vi "ReadSerialNumber.vi"(8 "error in (no error)":errorcluster, 11 "TestBench in":refnum<class "TestBench.lvclass">) -> (0 "error out":errorcluster, 3 "TestBench out":refnum<class "TestBench.lvclass">)   [LabVIEW 2019, in "TestBench.lvlib" / "TestBench.lvclass"]
uses:
  TestBench.lvclass
  TestBench.lvclass/TestBench.ctl
  TestEngine/TestEngine Messages/Write SerialNumber Msg/Write SerialNumber Msg.lvclass/Write SerialNumber Msg.ctl
  <vilib>/ActorFramework/Message Enqueuer/Message Enqueuer.lvclass/Message Enqueuer.ctl
  <vilib>/ActorFramework/Message Enqueuer/Enqueue.vi
  TestEngine/TestEngine Messages/Write SerialNumber Msg/Write SerialNumber Msg.lvclass
  C:/Program Files (x86)/National Instruments/LabVIEW 2019/vi.lib/ActorFramework/Message/Message.lvclass
  <vilib>/ActorFramework/Message Priority Queue/Priority Enqueue.vi
panel:
  in  "Cancel":bool
  in  "SerialNumber":string
  in  "OK":bool
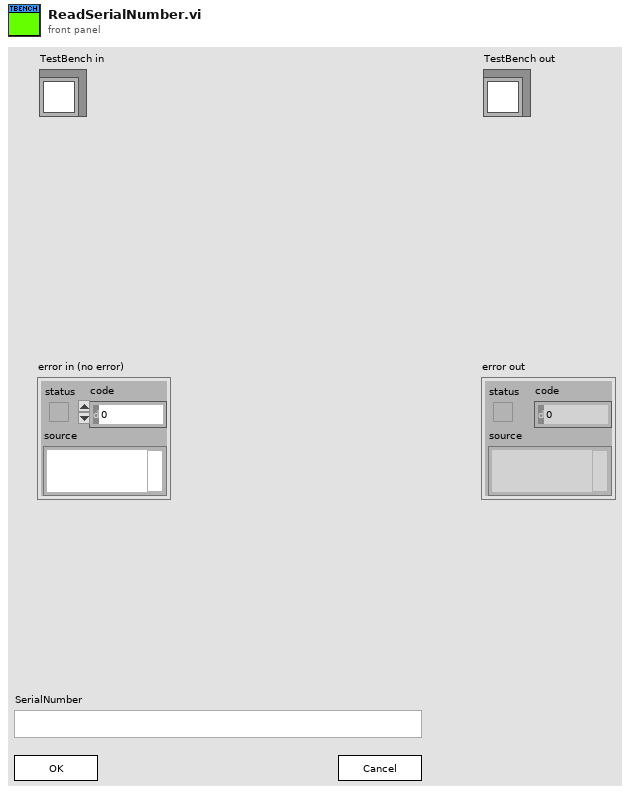
[diagram p1: front panel]
types:
  T1 = map{string, refnum<class "Message Enqueuer.lvclass">}
  T2 = cluster{string, "TestEngine Actor's Enqueuer":refnum<class "Message Enqueuer.lvclass">}
  T3 = enum32{"Invalid", "Standard", "Closed", "Hidden", "Minimized", "Maximized"}
  T4 = enum32{"invalid app kind", "Development System", "Run Time System", "Student Edition", "Embedded LabVIEW", "Evaluation", "Custom"}
  T5 = cluster{"Core":cluster{"Current VI Reference":refnum<vi>, "Close Panel on Exit?":bool}, "Your string data":string, "SerialNumber":refnum<vi>}
  T6 = cluster{"Current VI Reference":refnum<vi>, "Close Panel on Exit?":bool}
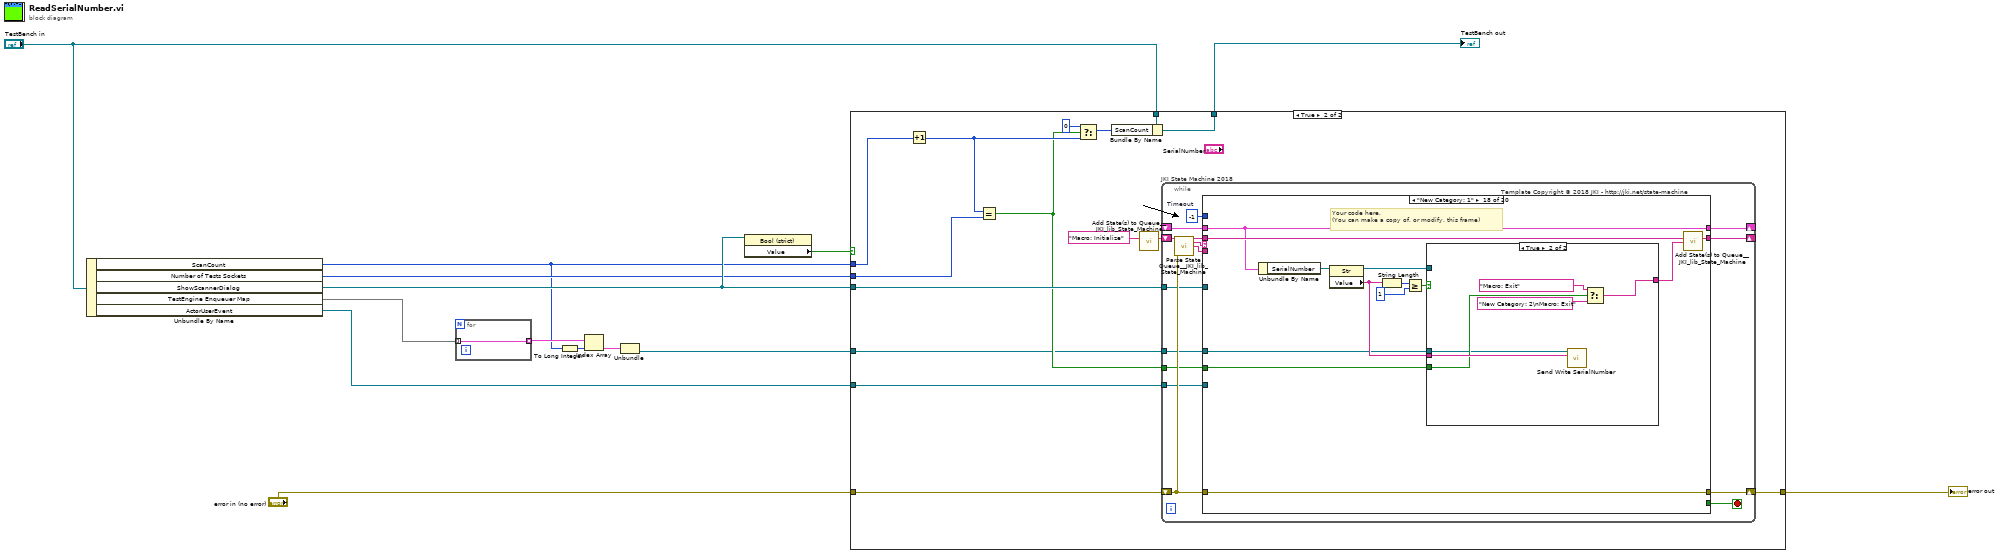
[diagram p0: block diagram]
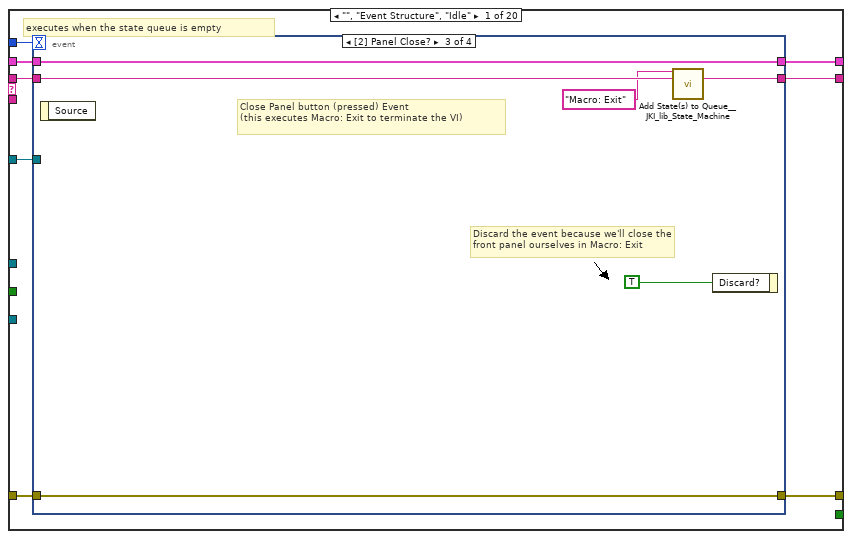
[diagram p3: hidden frame]
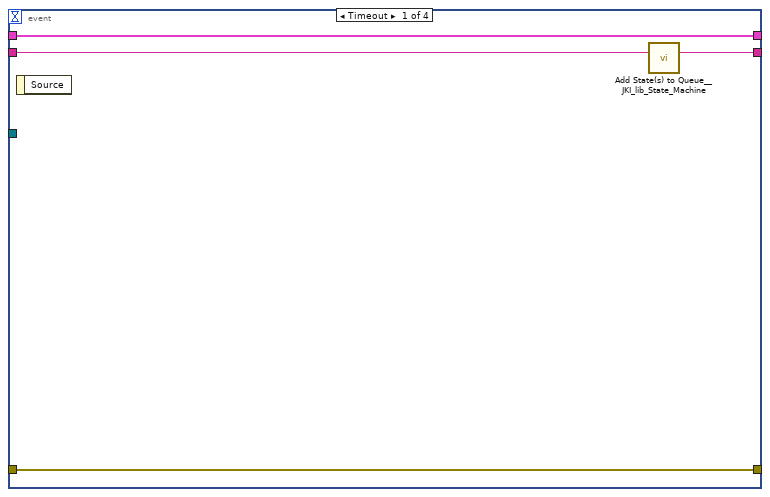
[diagram p4: hidden frame]
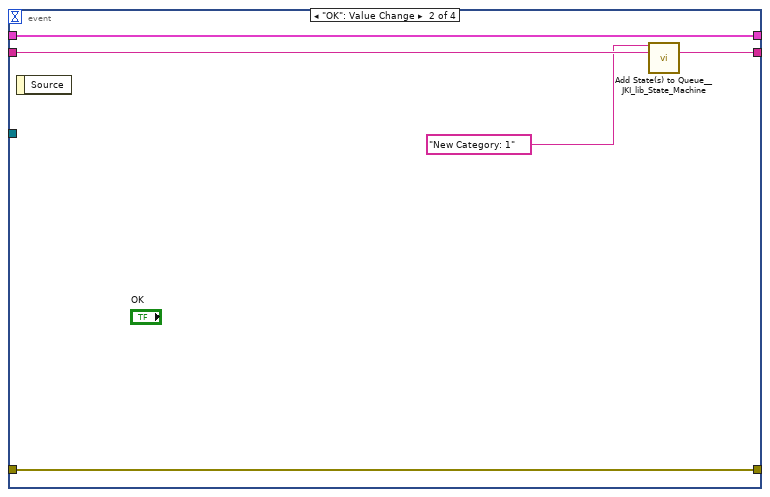
[diagram p5: hidden frame]
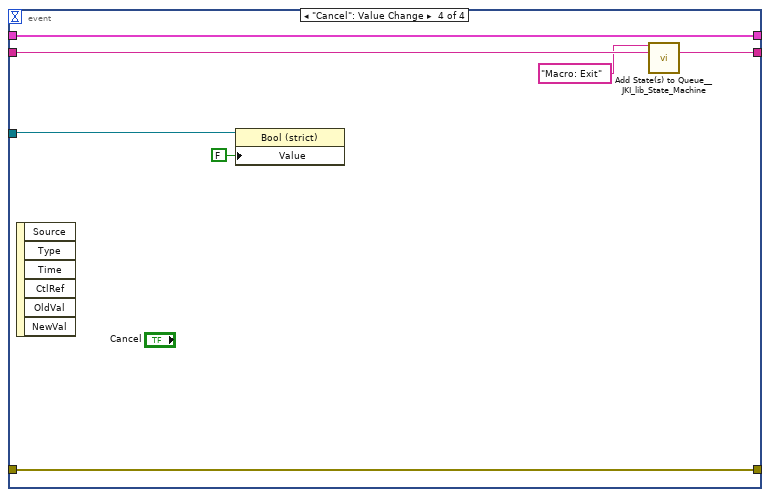
[diagram p6: hidden frame]
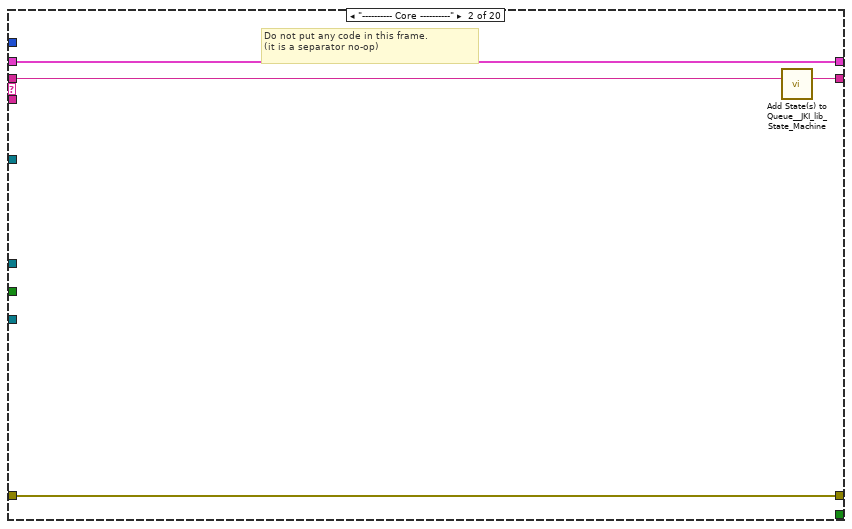
[diagram p7: hidden frame]
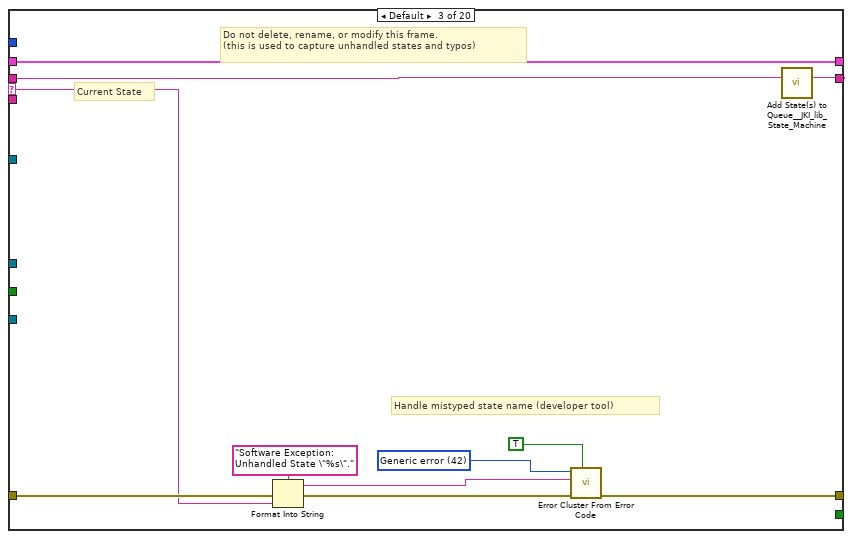
[diagram p8: hidden frame]
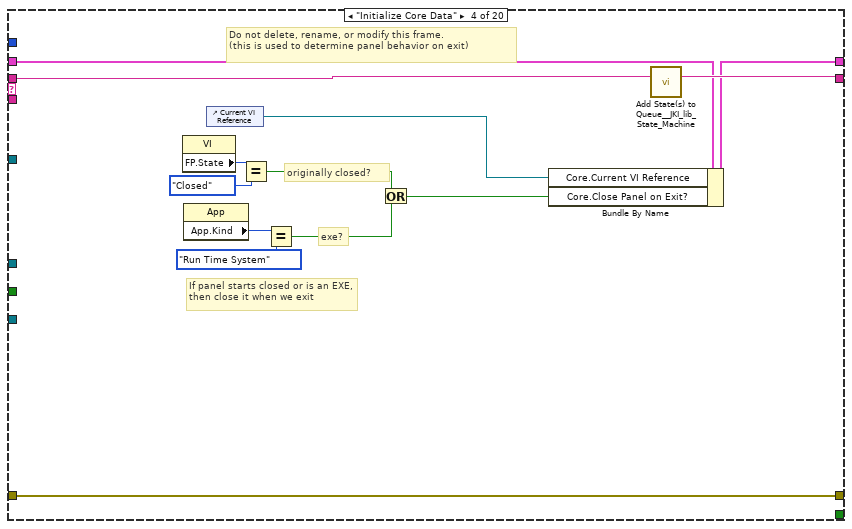
[diagram p9: hidden frame]
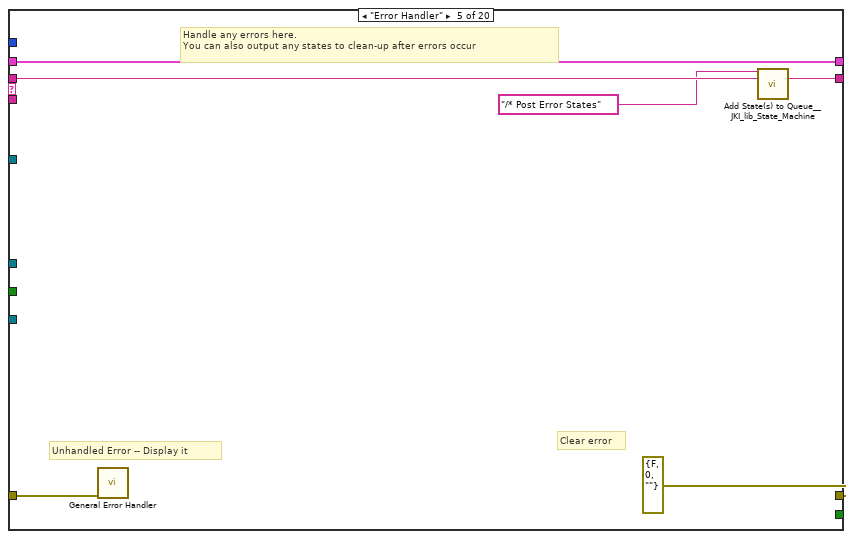
[diagram p10: hidden frame]
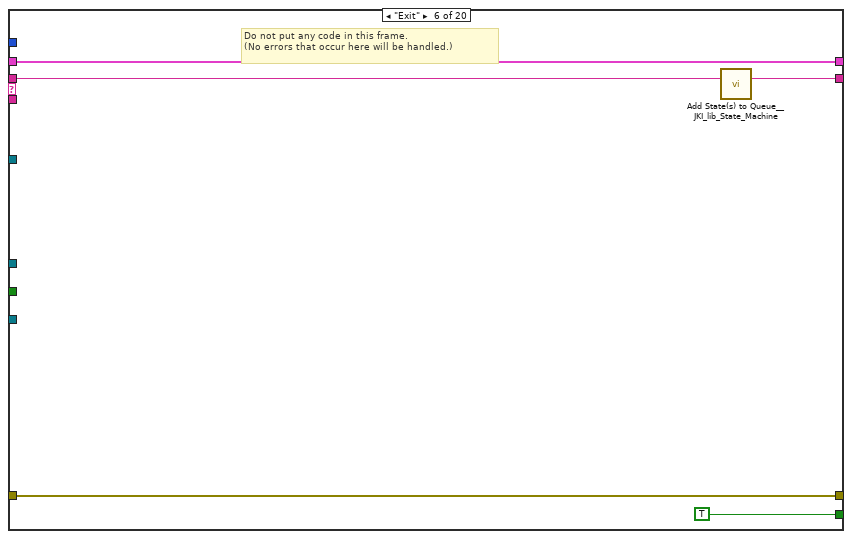
[diagram p11: hidden frame]
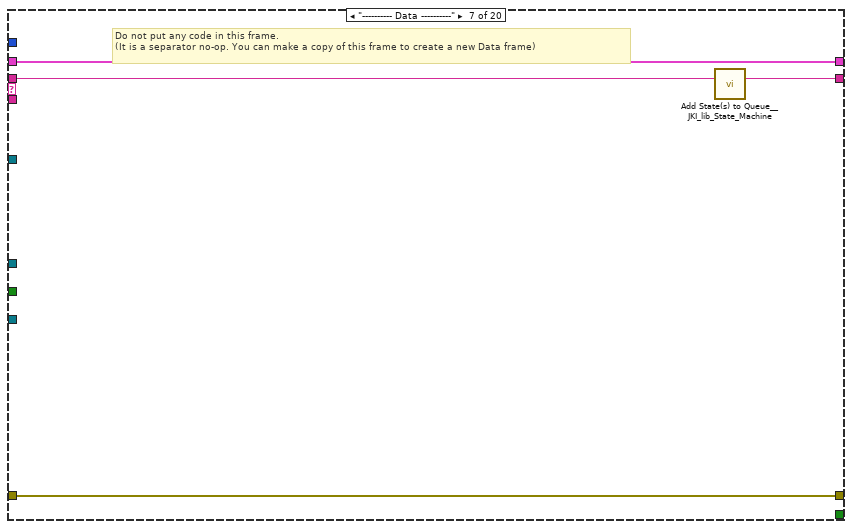
[diagram p12: hidden frame]
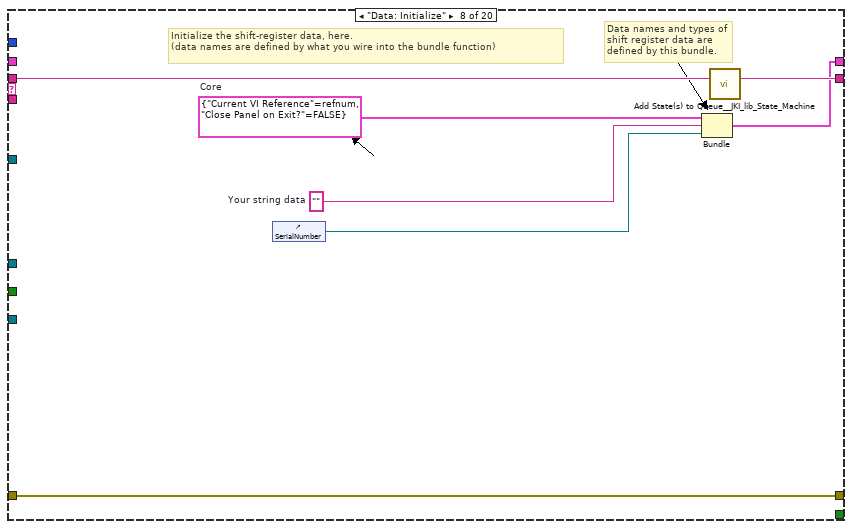
[diagram p13: hidden frame]
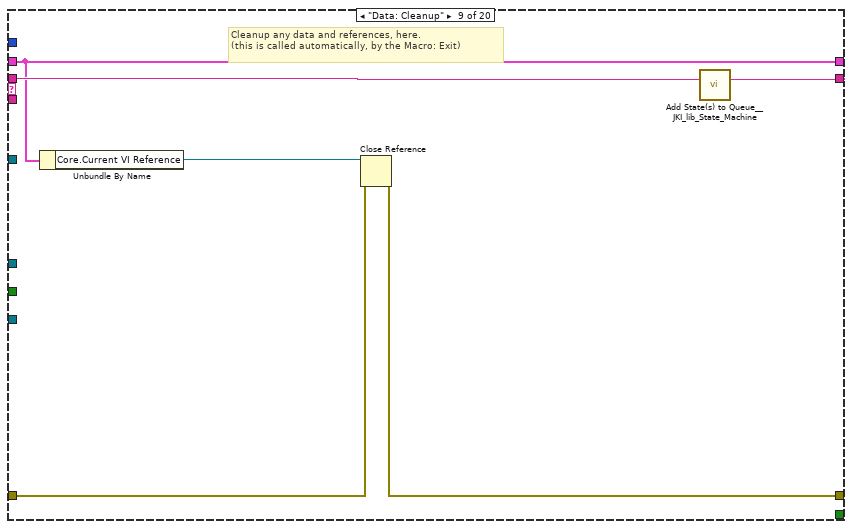
[diagram p14: hidden frame]
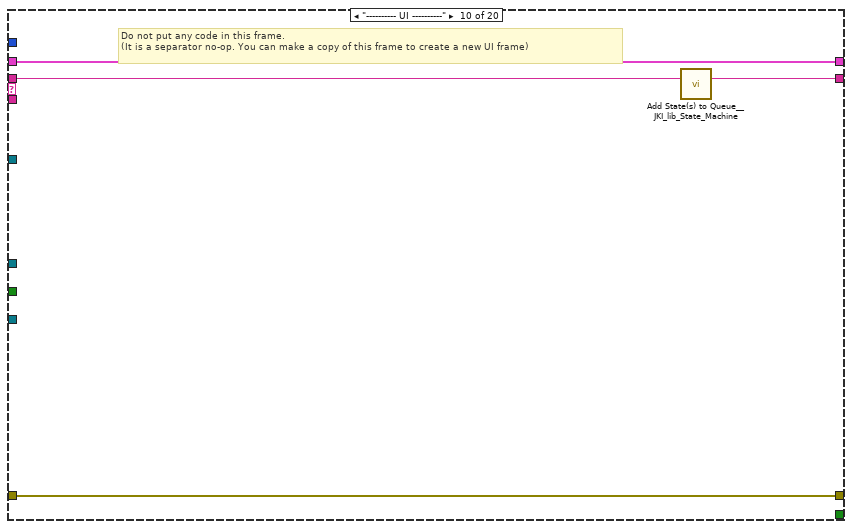
[diagram p15: hidden frame]
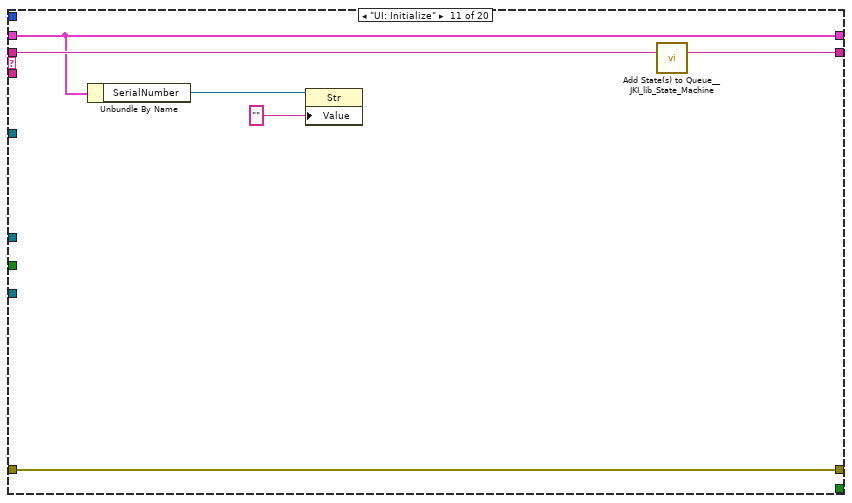
[diagram p16: hidden frame]
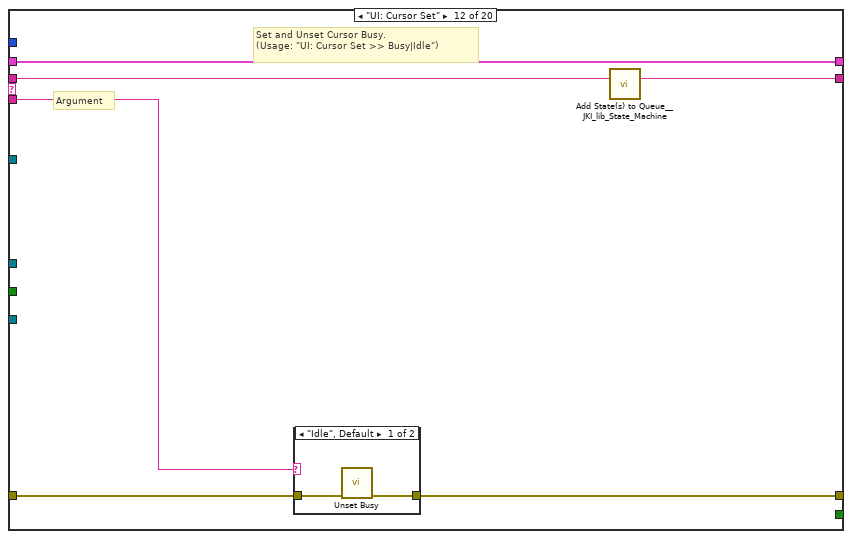
[diagram p17: hidden frame]
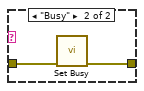
[diagram p18: hidden frame]
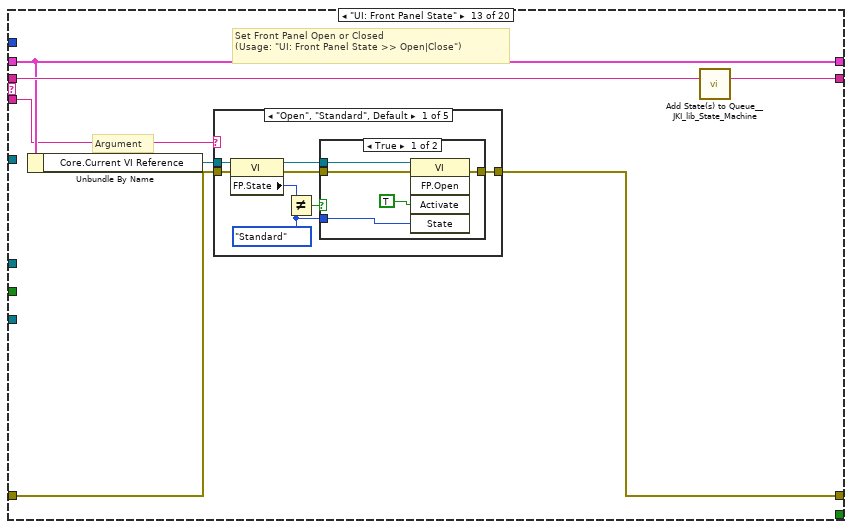
[diagram p19: hidden frame]
diagram:
  n1 = Unbundle By Name("TestBench in") -> ("ScanCount"=w4:u8, "Number of Tests Sockets"=w9:u8, "ShowScannerDialog"=w11:refnum<vi>, "TestEngine Enqueuer Map"=w6:T1, "ActorUserEvent"=w10:refnum<user-event>)
  n2 = for {
    tunnel: [w15] -> w5 mode=indexing
    tunnel: w6 -> [w15] mode=indexing
  }
  n3 = To Long Integer(number=w4) -> (32bit integer=w3:i32)
  n4 = Index Array(array=w5, index=w3) -> (element=w2:T2)
  n5 = Unbundle(w2) -> ("TestEngine Actor's Enqueuer"=w1:refnum<class "Message Enqueuer.lvclass">)  [unwired: 1 out]
  n6 = property class="Bool (strict)"(reference=w11) -> ("Value"=w12:bool)  [unwired: 1 in, 2 out]
  n7 = case shown="True" w12 {
    tunnel: "error in (no error)" -> [w17 w30]
    tunnel: [w17 w29] -> w13
    tunnel: w11 -> [_ w28]
    tunnel: w10 -> [_ w27]
    tunnel: w4 -> [_ w24]
    tunnel: w9 -> [_ w23]
    tunnel: "TestBench in" -> [w16 w20]
    tunnel: [w16 w19] -> w7
    tunnel: w1 -> [_ w18]
    frame False {
    }
    frame True {
      n8 = Increment(x=w24) -> (x+1=w26:u8)
      n9 = Equal?(x=w26, y=w23) -> (x = y?=w22:bool)
      n10 = Select(t=u8 0, s=w22, f=w26) -> (s? t:f=w21:u8)
      n11 = Bundle By Name(cluster=w20, "ScanCount"=w21) -> (w19:refnum<class "TestBench.lvclass">)
      n12 = call <vilib>:"Add State(s) to Queue__JKI_lib_State_Machine.vi"("State(s) in (\"\")"="Macro: Initialize") -> ("States Out"=w32:string)  [unwired: 14 in]
      n13 = while "JKI State Machine 2018" {
        shift-right: [w40] -> _
        shift-left: _ -> [w39]
        shift-right: [w43] -> w29
        shift-left: w30 -> [w37]
        shift-right: [w42] -> _
        shift-left: w32 -> [w44]
        tunnel: w28 -> [w36]
        tunnel: w27 -> [w35]
        tunnel: w22 -> [w34]
        tunnel: w18 -> [w33]
        stop <- w41 stop-if-true
        w38 = -1  # Timeout
        # "Template Copyright © 2018 JKI - http://jki.net/state-machine"
        n14 = call <vilib>:"Parse State Queue__JKI_lib_State_Machine.vi"("State Queue"=w44, "Error In (no error)"=w37) -> ("Remaining States"=w46:string, "Current State"=w47:string, "Arguments"=w45:string)  [unwired: 11 in]
        n15 = case shown="\"New Category: 1\"" w47 {
          selector: w47 -> [_ _ w82 _ _ _ _ _ _ _ _ _ _ _ _ _ _ _ _ _]
          tunnel: w46 -> [w55 w81 w86 w105 w111 w116 w120 w127 w133 w137 w143 w149 w160 w229 w234 w244 w248 w261 w279 w285]
          tunnel: w45 -> [_ _ _ _ _ _ _ _ _ _ _ w144 w154 _ _ _ _ _ _ _]
          tunnel: w39 -> [w53 w78 w84 w98 w108 w114 w117 _ w128 w134 w138 w147 w156 w226 w231 w241 w245 w258 w276 w281]
          tunnel: [w52 w79 w88 w102 errorcluster {"status"=FALSE, "code"=0, "source"=""} ("error out") w113 w118 w124 w129 w135 w141 w145 w157 w227 w232 w242 w246 w259 w277 w283] -> w43
          tunnel: w37 -> [w51 w79 w87 w102 w107 w113 w118 w124 w130 w135 w141 w146 w158 w227 w232 w242 w246 w259 w277 w283]
          tunnel: [w54 w80 w85 w104 w110 w115 w119 w126 w132 w136 w142 w148 w159 w228 w233 w243 w247 w260 w278 w284] -> w42
          tunnel: [_ _ _ _ _ TRUE _ _ _ _ _ _ _ _ _ _ _ _ _ _] -> w41
          tunnel: [w50 w78 w84 w103 w108 w114 w117 w125 w128 w134 w138 w147 w156 w226 w231 w241 w245 w258 w276 w281] -> w40
          tunnel: w38 -> [w49 _ _ _ _ _ _ _ _ _ _ _ _ _ _ _ _ _ _ _]
          tunnel: w36 -> [w48 _ _ _ _ _ _ _ _ _ _ _ _ _ _ _ _ _ _ _]
          tunnel: w35 -> [_ _ _ _ _ _ _ _ _ _ _ _ _ _ _ _ _ _ w275 _]
          tunnel: w34 -> [_ _ _ _ _ _ _ _ _ _ _ _ _ _ _ _ _ w251 _ _]
          tunnel: w33 -> [_ _ _ _ _ _ _ _ _ _ _ _ _ _ _ _ _ w249 _ _]
          frame "", "Event Structure", "Idle" {
            # "executes when the state queue is empty"
            n16 = event shown="[2] Panel Close?" {
              selector: _ -> [_ _ _ _]
              dyn-events: _ -> [_ _ _ _]
              timeout: w49 -> [_ _ _ _]
              tunnel: w55 -> [w59 w64 w70 w77]
              tunnel: [w58 w63 w69 w76] -> w54
              tunnel: w53 -> [w56 w61 w67 w74]
              tunnel: [w57 w62 w68 w75] -> w52
              tunnel: w51 -> [w57 w62 w68 w75]
              tunnel: [w56 w61 w67 w74] -> w50
              tunnel: w48 -> [_ _ _ w72]
              event Timeout {
                n17 = event-data() -> ()  [unwired: 1 in, 1 out]
                n18 = call <vilib>:"Add State(s) to Queue__JKI_lib_State_Machine.vi"("State(s) in (\"\")"=w59) -> ("States Out"=w58:string)  [unwired: 14 in]
              }
              event "OK": Value Change {
                n19 = event-data() -> ()  [unwired: 1 in, 1 out]
                n20 = call <vilib>:"Add State(s) to Queue__JKI_lib_State_Machine.vi"("State(s) in Front (\"\")"="New Category: 1", "State(s) in (\"\")"=w64) -> ("States Out"=w63:string)  [unwired: 13 in]
              }
              event Panel Close? {
                # "Discard the event because we'll close the front panel ourselves in Macro: Exit"
                # "Close Panel button (pressed) Event\n(this executes Macro: Exit to terminate the VI)"
                n21 = event-data() -> ()  [unwired: 1 in, 1 out]
                n22 = call <vilib>:"Add State(s) to Queue__JKI_lib_State_Machine.vi"("State(s) in Front (\"\")"="Macro: Exit", "State(s) in (\"\")"=w70) -> ("States Out"=w69:string)  [unwired: 13 in]
                n23 = event-data("Discard?"=TRUE) -> ()  [unwired: 1 in, 1 out]
              }
              event "Cancel": Value Change {
                n24 = event-data() -> ()  [unwired: 1 in, 6 out]
                n25 = property class="Bool (strict)"(reference=w72, "Value"=FALSE) -> ()  [unwired: 1 in, 2 out]
                n26 = call <vilib>:"Add State(s) to Queue__JKI_lib_State_Machine.vi"("State(s) in Front (\"\")"="Macro: Exit", "State(s) in (\"\")"=w77) -> ("States Out"=w76:string)  [unwired: 13 in]
              }
            }
          }
          frame "---------- Core ----------" {
            # "Do not put any code in this frame.\n(it is a separator no-op)"
            n27 = call <vilib>:"Add State(s) to Queue__JKI_lib_State_Machine.vi"("State(s) in (\"\")"=w81) -> ("States Out"=w80:string)  [unwired: 14 in]
          }
          frame Default {
            w91 = 42 items=["No error", "Argument error", "Memory is full", "Out of zone", "End of file", "File already open", "Generic file I/O error", "File not found", "File permission error", "Disk is full", "Duplicate path", "Too many files open", "System feature not enabled", "Resource file not found", "Cannot add resource", "Resource not found", "Image not found", "Image memory error", "Pen does not exist", "Config type invalid", "Config token not found", "Config parse error", "Config memory error", "Bad external code format", "Bad external code offset", "External code not present", "Null window", "Destroy window error", "Null menu", "Print aborted", "Bad print record", "Print driver error", "Windows error during printing", "Memory error during printing", "Print dialog error", "Generic print error", "Invalid device refnum", "Device not found", "Device parameter error", "Device unit error", "Cannot open device", "Device call aborted", "Generic error", "Cancelled by user", "Object ID too low", "Object ID too high", "Object not in heap", "Unknown heap", "Unknown object (invalid DefProc)", "Unknown object (DefProc not in table)", "Message out of range", "Invalid (null) method", "Unknown message", "Manager call not supported", "Bad address", "Network operation in progress", "Network operation timed out", "Connection is busy", "Network attribute not supported", "Network error", "Address in use", "System out of memory", "Connection aborted", "Connection refused", "Not connected", "Already connected", "Connection closed", "Initialization error (interapplication manager)", "Bad occurrence", "Wait on unbound occurrence handler", "Occurrence queue overflow", "Datalog type conflict", "Unused", "Unrecognized type (interapplication manager)", "Memory corrupt", "Failed to make temporary DLL", "Old CIN version", "Drag socket not found", "Failed to load drop-object", "Failed to register OLE object", "Failed to release OLE object", "Format specifier type mismatch", "Unknown format specifier", "Too few format specifiers", "Too many format specifiers", "Scan failed", "Newer CIN version", "Error converting to variant", "Runtime menu error", "Password tampered", "Variant attribute not found", "Incompatible variant data type", "Event data is not available", "Event Store is not present", "Occurrence is not found", "Event Queue is not created", "Event info is not available", "Refnum passed is NULL", "Error retrieving Class GUID", "Error retrieving CoClass GUID", "Error retrieving TypeLib GUID.", "Bad built application magic bytes.", "Specific driver is different from the specific driver associated with the Logical Name.", "There is no session opened to the class driver.", "Max Error", "MAX - Error with config objects", "MAX - Error loading configuration", "MAX - Group not supported"]
            # "Current State"
            # "Do not delete, rename, or modify this frame.\n(this is used to capture unhandled states and typos)"
            # "Handle mistyped state name (developer tool)"
            n28 = Format Into String(format string="Software Exception: Unhandled State \"%s\"." ("message"), error in=w87, w82) -> (resulting string=w90:string, error out=w89:errorcluster)  [unwired: 1 in]
            n29 = call <vilib>:"Error Cluster From Error Code.vi"("show call chain? (False)"=TRUE, "error in (no error)"=w89, "error message (\"\")"=w90, "error code (0)"=w91) -> ("error out"=w88:errorcluster)  [unwired: 5 in]
            n30 = call <vilib>:"Add State(s) to Queue__JKI_lib_State_Machine.vi"("State(s) in (\"\")"=w86) -> ("States Out"=w85:string)  [unwired: 14 in]
          }
          frame "Initialize Core Data" {
            # "Do not delete, rename, or modify this frame.\n(this is used to determine panel behavior on exit)"
            # "originally closed?"
            # "exe?"
            # "If panel starts closed or is an EXE, then close it when we exit"
            n31 = property class="VI"() -> ("FP.State"=w95:T3)  [unwired: 2 in, 2 out]
            n32 = property class="App"() -> ("App.Kind"=w101:T4)  [unwired: 2 in, 2 out]
            n33 = control-ref of="Current VI Reference"() -> (w96:refnum<vi>)
            n34 = Equal?(x=w95, y=T3."Closed" ("Front Panel Window:State")) -> (x = y?=w93:bool)
            n35 = Equal?(x=w101, y=T4."Run Time System" ("Application:Kind")) -> (x = y?=w99:bool)
            n36 = Or(x=w93, y=w99) -> (x .or. y?=w97:bool)
            n37 = Bundle By Name(cluster=w98, "Core.Current VI Reference"=w96, "Core.Close Panel on Exit?"=w97) -> (w103:T5)
            n38 = call <vilib>:"Add State(s) to Queue__JKI_lib_State_Machine.vi"("State(s) in (\"\")"=w105) -> ("States Out"=w104:string)  [unwired: 14 in]
          }
          frame "Error Handler" {
            # "Unhandled Error -- Display it"
            # "Handle any errors here.\nYou can also output any states to clean-up after errors occur"
            # "Clear error"
            n39 = call <vilib>:"General Error Handler.vi"("error in (no error)"=w107) -> ()  [unwired: 10 in, 5 out]
            n40 = call <vilib>:"Add State(s) to Queue__JKI_lib_State_Machine.vi"("State(s) in Front (\"\")"="/* Post Error States", "State(s) in (\"\")"=w111) -> ("States Out"=w110:string)  [unwired: 13 in]
          }
          frame "Exit" {
            # "Do not put any code in this frame.\n(No errors that occur here will be handled.)"
            n41 = call <vilib>:"Add State(s) to Queue__JKI_lib_State_Machine.vi"("State(s) in (\"\")"=w116) -> ("States Out"=w115:string)  [unwired: 14 in]
          }
          frame "---------- Data ----------" {
            # "Do not put any code in this frame.\n(It is a separator no-op. You can make a copy of this frame to create a new Data frame)"
            n42 = call <vilib>:"Add State(s) to Queue__JKI_lib_State_Machine.vi"("State(s) in (\"\")"=w120) -> ("States Out"=w119:string)  [unwired: 14 in]
          }
          frame "Data: Initialize" {
            w123 = T6 {"Current VI Reference"=refnum, "Close Panel on Exit?"=FALSE}  # Core
            w121 = ""  # Your string data
            # "Data names and types of shift register data are defined by this bundle."
            # "Initialize the shift-register data, here.\n(data names are defined by what you wire into the bundle function)"
            n43 = control-ref of="SerialNumber"() -> (w122:refnum<vi>)
            n44 = Bundle("Core"=w123, "Your string data"=w121, "SerialNumber"=w122) -> (w125:T5)  [unwired: 1 in]
            n45 = call <vilib>:"Add State(s) to Queue__JKI_lib_State_Machine.vi"("State(s) in (\"\")"=w127) -> ("States Out"=w126:string)  [unwired: 14 in]
          }
          frame "Data: Cleanup" {
            # "Cleanup any data and references, here.\n(this is called automatically, by the Macro: Exit)"
            n46 = Unbundle By Name(w128) -> ("Core.Current VI Reference"=w131:refnum<vi>)
            n47 = Close Reference(reference=w131, error in (no error)=w130) -> (error out=w129:errorcluster)
            n48 = call <vilib>:"Add State(s) to Queue__JKI_lib_State_Machine.vi"("State(s) in (\"\")"=w133) -> ("States Out"=w132:string)  [unwired: 14 in]
          }
          frame "---------- UI ----------" {
            # "Do not put any code in this frame.\n(It is a separator no-op. You can make a copy of this frame to create a new UI frame)"
            n49 = call <vilib>:"Add State(s) to Queue__JKI_lib_State_Machine.vi"("State(s) in (\"\")"=w137) -> ("States Out"=w136:string)  [unwired: 14 in]
          }
          frame "UI: Initialize" {
            n50 = Unbundle By Name(w138) -> ("SerialNumber"=w140:refnum<vi>)
            n51 = property class="Str"(reference=w140, "Value"="") -> ()  [unwired: 1 in, 2 out]
            n52 = call <vilib>:"Add State(s) to Queue__JKI_lib_State_Machine.vi"("State(s) in (\"\")"=w143) -> ("States Out"=w142:string)  [unwired: 14 in]
          }
          frame "UI: Cursor Set" {
            # "Argument"
            # "Set and Unset Cursor Busy.\n(Usage: \"UI: Cursor Set >> Busy|Idle\")"
            n53 = case shown="\"Idle\", Default" w144 {
              tunnel: w146 -> [w151 w153]
              tunnel: [w150 w152] -> w145
              frame "Idle", Default {
                n54 = call <vilib>:"Unset Busy.vi"("error in (no error)"=w151) -> ("error out"=w150:errorcluster)  [unwired: 10 in]
              }
              frame "Busy" {
                n55 = call <vilib>:"Set Busy.vi"("error in (no error)"=w153) -> ("error out"=w152:errorcluster)  [unwired: 9 in, 1 out]
              }
            }
            n56 = call <vilib>:"Add State(s) to Queue__JKI_lib_State_Machine.vi"("State(s) in (\"\")"=w149) -> ("States Out"=w148:string)  [unwired: 14 in]
          }
          frame "UI: Front Panel State" {
            # "Argument"
            # "Set Front Panel Open or Closed\n(Usage: \"UI: Front Panel State >> Open|Close\")"
            n57 = Unbundle By Name(w156) -> ("Core.Current VI Reference"=w155:refnum<vi>)
            n58 = case shown="\"Open\", \"Standard\", Default" w154 {
              tunnel: w158 -> [w166 w181 w192 w205 w218]
              tunnel: [w168 w182 w194 w207 w220] -> w157
              tunnel: w155 -> [w167 w179 w193 w206 w219]
              frame "Open", "Standard", Default {
                w161 = T3."Standard" ("State")
                n59 = property class="VI"(reference=w167, error in=w166) -> (reference out=w164:refnum<vi>, error out=w165:errorcluster, "FP.State"=w163:T3)
                n60 = Not Equal?(x=w163, y=w161) -> (x != y?=w162:bool)
                n61 = case shown="True" w162 {
                  tunnel: [w172 w174] -> w168
                  tunnel: w165 -> [w171 w174]
                  tunnel: w164 -> [w170 _]
                  tunnel: w161 -> [w169 _]
                  frame True {
                    n62 = invoke class="VI" method="FP.Open"(reference=w170, error in=w171, "Activate"=TRUE, "State"=w169) -> (error out=w172:errorcluster)  [unwired: 1 in, 4 out]
                  }
                  frame False {
                  }
                }
              }
              frame "Close", "Closed" {
                n63 = property class="VI"(reference=w179, error in=w181) -> (reference out=w178:refnum<vi>, error out=w180:errorcluster, "FP.State"=w176:T3)
                n64 = Not Equal?(x=w176, y=T3."Closed" ("Front Panel Window:State")) -> (x != y?=w175:bool)
                n65 = case shown="True" w175 {
                  tunnel: [w183 w186] -> w182
                  tunnel: w180 -> [w183 w185]
                  tunnel: w178 -> [_ w184]
                  frame False {
                  }
                  frame True {
                    n66 = invoke class="VI" method="FP.Close"(reference=w184, error in=w185) -> (error out=w186:errorcluster)  [unwired: 1 in, 2 out]
                  }
                }
              }
              frame "Hidden", "Hide" {
                w187 = T3."Hidden" ("State")
                n67 = property class="VI"(reference=w193, error in=w192) -> (reference out=w190:refnum<vi>, error out=w191:errorcluster, "FP.State"=w189:T3)
                n68 = Not Equal?(x=w189, y=w187) -> (x != y?=w188:bool)
                n69 = case shown="True" w188 {
                  tunnel: [w198 w199] -> w194
                  tunnel: w191 -> [w197 w199]
                  tunnel: w190 -> [w196 _]
                  tunnel: w187 -> [w195 _]
                  frame True {
                    n70 = invoke class="VI" method="FP.Open"(reference=w196, error in=w197, "State"=w195) -> (error out=w198:errorcluster)  [unwired: 2 in, 4 out]
                  }
                  frame False {
                  }
                }
              }
              frame "Minimize", "Minimized" {
                w200 = T3."Minimized" ("State")
                n71 = property class="VI"(reference=w206, error in=w205) -> (reference out=w203:refnum<vi>, error out=w204:errorcluster, "FP.State"=w202:T3)
                n72 = Not Equal?(x=w202, y=w200) -> (x != y?=w201:bool)
                n73 = case shown="True" w201 {
                  tunnel: [w211 w212] -> w207
                  tunnel: w204 -> [w210 w212]
                  tunnel: w203 -> [w209 _]
                  tunnel: w200 -> [w208 _]
                  frame True {
                    n74 = invoke class="VI" method="FP.Open"(reference=w209, error in=w210, "State"=w208) -> (error out=w211:errorcluster)  [unwired: 2 in, 4 out]
                  }
                  frame False {
                  }
                }
              }
              frame "Maximize", "Maximized" {
                w213 = T3."Maximized" ("State")
                n75 = property class="VI"(reference=w219, error in=w218) -> (reference out=w216:refnum<vi>, error out=w217:errorcluster, "FP.State"=w215:T3)
                n76 = Not Equal?(x=w215, y=w213) -> (x != y?=w214:bool)
                n77 = case shown="True" w214 {
                  tunnel: [w224 w225] -> w220
                  tunnel: w217 -> [w223 w225]
                  tunnel: w216 -> [w222 _]
                  tunnel: w213 -> [w221 _]
                  frame True {
                    n78 = invoke class="VI" method="FP.Open"(reference=w222, error in=w223, "State"=w221) -> (error out=w224:errorcluster)  [unwired: 2 in, 4 out]
                  }
                  frame False {
                  }
                }
              }
            }
            n79 = call <vilib>:"Add State(s) to Queue__JKI_lib_State_Machine.vi"("State(s) in (\"\")"=w160) -> ("States Out"=w159:string)  [unwired: 14 in]
          }
          frame "---------- Macro ----------" {
            # "Do not put any code in this frame.\n(It is a separator no-op. You can make a copy of this frame to create a new Macro frame)"
            n80 = call <vilib>:"Add State(s) to Queue__JKI_lib_State_Machine.vi"("State(s) in (\"\")"=w229) -> ("States Out"=w228:string)  [unwired: 14 in]
          }
          frame "Macro: Initialize" {
            w230 = "Data: Initialize\nInitialize Core Data\nUI: Initialize\nUI: Front Panel State >> Open\nNew Category: 3"  # Data: Initialize Initialize Core Data UI: Initialize UI: Front Panel State >> Open New Category: 3
            # "Initialization Macro\n(This is called once, when the VI starts)"
            n81 = call <vilib>:"Add State(s) to Queue__JKI_lib_State_Machine.vi"("State(s) in Front (\"\")"=w230, "State(s) in (\"\")"=w234) -> ("States Out"=w233:string)  [unwired: 13 in]
          }
          frame "Macro: Exit" {
            # "Exit Macro\n(This is called once, when the VI exits)"
            n82 = Unbundle By Name(w241) -> ("Core.Close Panel on Exit?"=w240:bool)
            n83 = Select(t="UI: Front Panel State >> Close", s=w240, f="") -> (s? t:f=w237:string)
            n84 = call <vilib>:"Add State(s) to Queue__JKI_lib_State_Machine.vi"("State(s) in (\"\")"=w237, "State(s) at Back (\"\")"="Data: Cleanup\nExit") -> ("States Out"=w235:string)  [unwired: 13 in]
            n85 = call <vilib>:"Add State(s) to Queue__JKI_lib_State_Machine.vi"("State(s) in Front (\"\")"=w235, "State(s) in (\"\")"=w244) -> ("States Out"=w243:string)  [unwired: 13 in]
          }
          frame "---------- New Category ----------" {
            # "Template Separator\n(You can make a copy of, or modify, this frame)"
            n86 = call <vilib>:"Add State(s) to Queue__JKI_lib_State_Machine.vi"("State(s) in (\"\")"=w248) -> ("States Out"=w247:string)  [unwired: 14 in]
          }
          frame "New Category: 1" {
            # "Your code here.\n(You can make a copy of, or modify, this frame)"
            n87 = Unbundle By Name(w258) -> ("SerialNumber"=w257:refnum<vi>)
            n88 = property class="Str"(reference=w257) -> (reference out=w252:refnum<vi>, "Value"=w253:string)  [unwired: 1 in, 1 out]
            n89 = String Length(string=w253) -> (length=w256:i32)
            n90 = Greater Or Equal?(x=w256, y=1) -> (x >= y?=w254:bool)
            n91 = case shown="True" w254 {
              tunnel: w253 -> [_ w273]
              tunnel: w252 -> [w263 _]
              tunnel: w251 -> [_ w271]
              tunnel: [_ w272] -> w250
              tunnel: w249 -> [_ w268]
              frame False {
                n92 = One Button Dialog(message="SerialNmuber Unqualified!") -> (true=w262:bool)  [unwired: 1 in]
                n93 = case shown="True" w262 {
                  tunnel: w263 -> [_ w267]
                  frame False {
                  }
                  frame True {
                    n94 = property class="Str"(reference=w267, "Value"="", "Key Focus"=TRUE) -> ()  [unwired: 1 in, 2 out]
                  }
                }
              }
              frame True {
                n95 = call "Send Write SerialNumber.vi"("SerialNumber"=w273, "Message Enqueuer"=w268) -> ()  [unwired: 8 in, 2 out]
                n96 = Select(t="Macro: Exit" ("State(s) at Back (\"\")"), s=w271, f="New Category: 2\nMacro: Exit" ("State(s) at Back (\"\")")) -> (s? t:f=w272:string)
              }
            }
            n97 = call <vilib>:"Add State(s) to Queue__JKI_lib_State_Machine.vi"("State(s) in (\"\")"=w261, "State(s) at Back (\"\")"=w250) -> ("States Out"=w260:string)  [unwired: 13 in]
          }
          frame "New Category: 2" {
            # "Your code here.\n(You can make a copy of, or modify, this frame)"
            n98 = Generate User Event(user event=w275, event data cluster=cluster{"Massage":string} {"Massage"="ReadSerialNumber"} ("event data")) -> ()  [unwired: 2 in, 2 out]
            n99 = call <vilib>:"Add State(s) to Queue__JKI_lib_State_Machine.vi"("State(s) in (\"\")"=w279) -> ("States Out"=w278:string)  [unwired: 14 in]
          }
          frame "New Category: 3" {
            # "Your code here.\n(You can make a copy of, or modify, this frame)"
            n100 = Unbundle By Name(w281) -> ("SerialNumber"=w280:refnum<vi>)
            n101 = property class="Str"(reference=w280, "Key Focus"=TRUE) -> ()  [unwired: 1 in, 2 out]
            n102 = call <vilib>:"Add State(s) to Queue__JKI_lib_State_Machine.vi"("State(s) in (\"\")"=w285) -> ("States Out"=w284:string)  [unwired: 14 in]
          }
        }
      }
    }
  }
  "error out" <- w13
  "TestBench out" <- w7
